vi "Set Initialize Edit Test Node.vi"(8 "error in (no error)":errorcluster, 10 "Initialize Edit Test Node":bool, 11 "Abstract Initialize Edit Test Node Msg in":refnum<class "Abstract Initialize Edit Test Node Msg.lvclass">) -> (0 "error out":errorcluster, 3 "Abstract Initialize Edit Test Node Msg out":refnum<class "Abstract Initialize Edit Test Node Msg.lvclass">)   [LabVIEW 2013, in "Edit Test Node Model.lvlib" / "Abstract Initialize Edit Test Node Msg.lvclass"]
uses:
  Abstract Initialize Edit Test Node Msg.lvclass
  Abstract Initialize Edit Test Node Msg.lvclass/Abstract Initialize Edit Test Node Msg.ctl
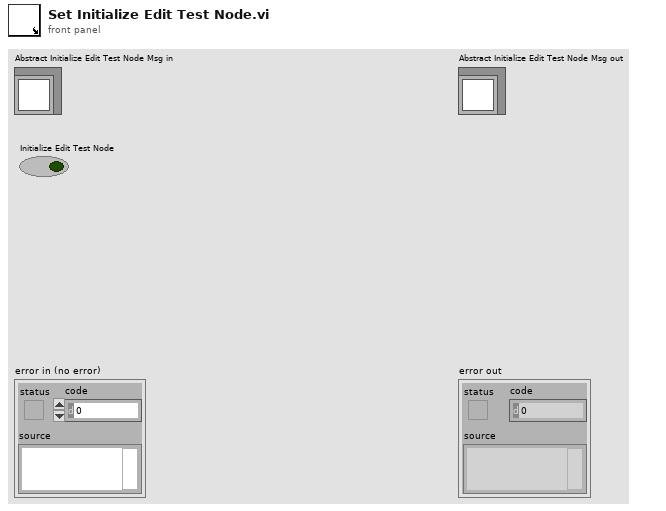
[diagram p1: front panel]
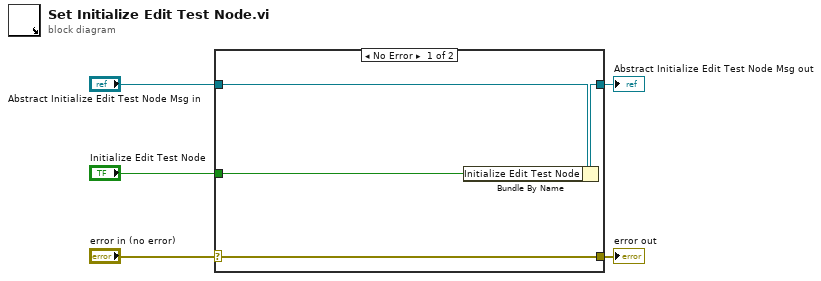
[diagram p0: block diagram]
diagram:
  n1 = case shown="No Error" "error in (no error)" {
    selector: "error in (no error)" -> [w9 w10]
    tunnel: [w9 w10] -> w4
    tunnel: [w7 w11] -> w2
    tunnel: "Abstract Initialize Edit Test Node Msg in" -> [w8 w11]
    tunnel: "Initialize Edit Test Node" -> [w6 _]
    frame No Error {
      n2 = Bundle By Name(cluster=w8, "Initialize Edit Test Node"=w6) -> (w7:refnum<class "Abstract Initialize Edit Test Node Msg.lvclass">)
    }
    frame Error {
    }
  }
  "error out" <- w4
  "Abstract Initialize Edit Test Node Msg out" <- w2
